vi "Get Password.vi"(8 "error in":errorcluster, 11 "password":string="admin") -> (0 "error out":errorcluster, 3 "Success?":bool)   [LabVIEW 2014]
panel:
  in  "OK Button":bool
  in  "input":string
  # "Please Enter Password"
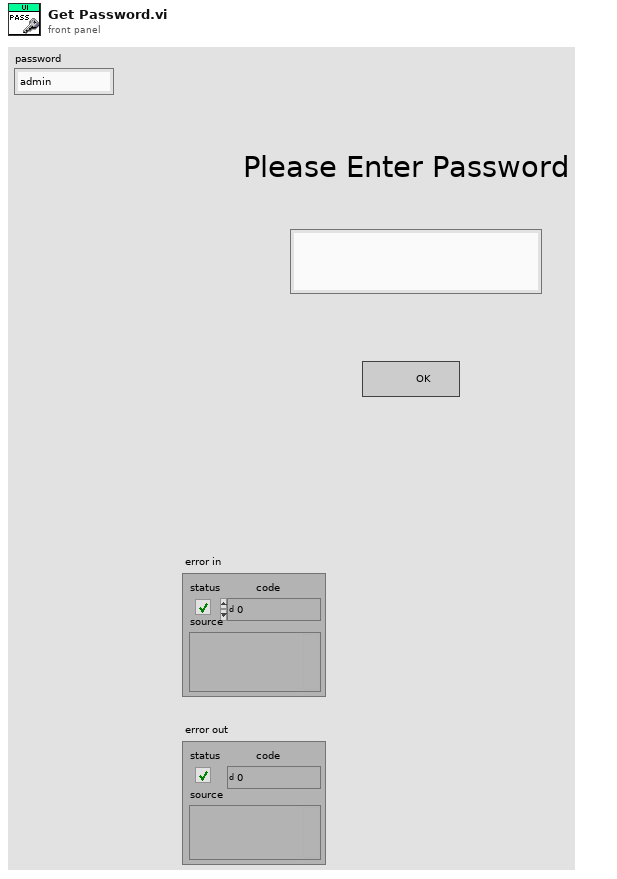
[diagram p1: front panel]
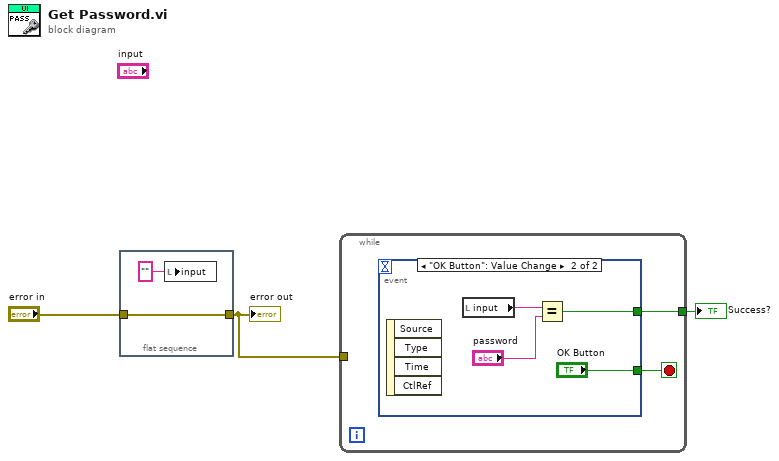
[diagram p0: block diagram]
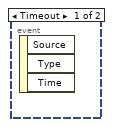
[diagram p2: hidden frame]
diagram:
  n1 = flat-sequence {
    tunnel: "error in" -> [w4]
    tunnel: [w4] -> w2
    frame #0 {
      n2 = local write "input"("" ("String")) -> ()
    }
  }
  n3 = while {
    tunnel: w2 -> [_]
    tunnel: [w6] -> w1
    stop <- w7 stop-if-true
    n4 = event shown="[1] \"OK Button\": Value Change" {
      selector: _ -> [_ _]
      dyn-events: _ -> [_ _]
      timeout: _ -> [_ _]
      tunnel: [_ "OK Button"] -> w7
      tunnel: [_ w9] -> w6
      event Timeout {
        n5 = event-data() -> ()  [unwired: 1 in, 3 out]
      }
      event "OK Button": Value Change {
        n6 = event-data() -> ()  [unwired: 1 in, 4 out]
        n7 = local read "input"() -> (w10:string)
        n8 = Equal?(x=w10, y="password") -> (x = y?=w9:bool)
      }
    }
  }
  "Success?" <- w1
  "error out" <- w2
